vi "ArmSimulatorReal.vi"() -> ()   [LabVIEW 2020]
uses:
  <vilib>/robotics/Kinematics/Plotting/NI_Robotics_3DKinematics.lvlib
  <vilib>/picture/3D Picture Control/NI_3D Picture Control.lvlib
  <vilib>/picture/3D Picture Control/Object/Add Object (no reference).vi
  <vilib>/robotics/Kinematics/NI_Kinematics.lvlib
  <vilib>/Utility/miscctls.llb/LV3DPointTypeDef.ctl
  a5137bdd-6b26-409e-be81-2a36b3426dbb.vi
  <vilib>/robotics/Kinematics/Robot/Forward Kinematics (Point).vi
  de8be538-574b-4146-99e0-83cb54bb3f19.vi
  <vilib>/robotics/Kinematics/dyn/Gravity Loading (Point).vi
  <vilib>/picture/3D Picture Control/Object/Create Object (drawable).vi
  <vilib>/Analysis/Matrix/Datatypes/RealMatrix.ctl
  <vilib>/Analysis/Matrix/NI_Matrix.lvlib
panel:
  in  "Angle":dbl
  out "torques":dbl[](array[numeric]) format="%.2f"
  out "end effector transform":T1
  out "Steps Taken":i32
  in  "Reset 3D View":bool
  out "IK Error":errorcluster
  in  "Goal Z (in)":dbl=28.0
  in  "Goal X (in)":dbl=-33.0
  out "3D Arm Simulation":refnum<vi>(3d-picture)
  # "<-- DOWN FIELD              SCORING GRID -->"
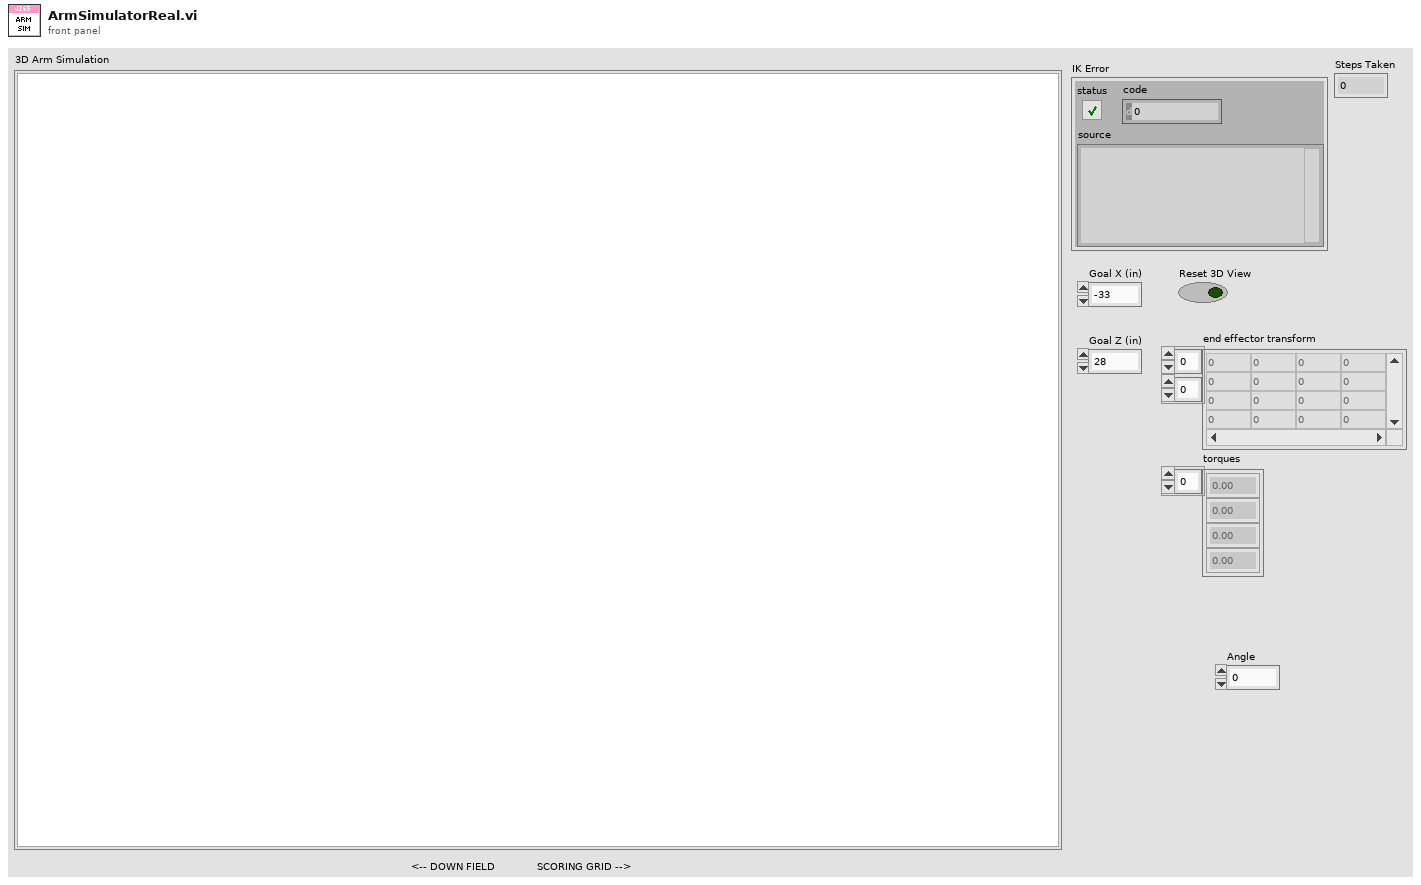
[diagram p1: front panel]
types:
  T1 = typedef "NI_Matrix.lvlib/RealMatrix.ctl" = dbl[][]
  T2 = cluster{"Red":sgl, "Green":sgl, "Blue":sgl, "Alpha":sgl}
  T3 = typedef "LV3DPointTypeDef.ctl" = cluster{"X":sgl, "Y":sgl, "Z":sgl}
  T4 = cluster{"Goal X (in)":dbl, "Goal Y (in)":dbl, "Goal Z (in)":dbl}
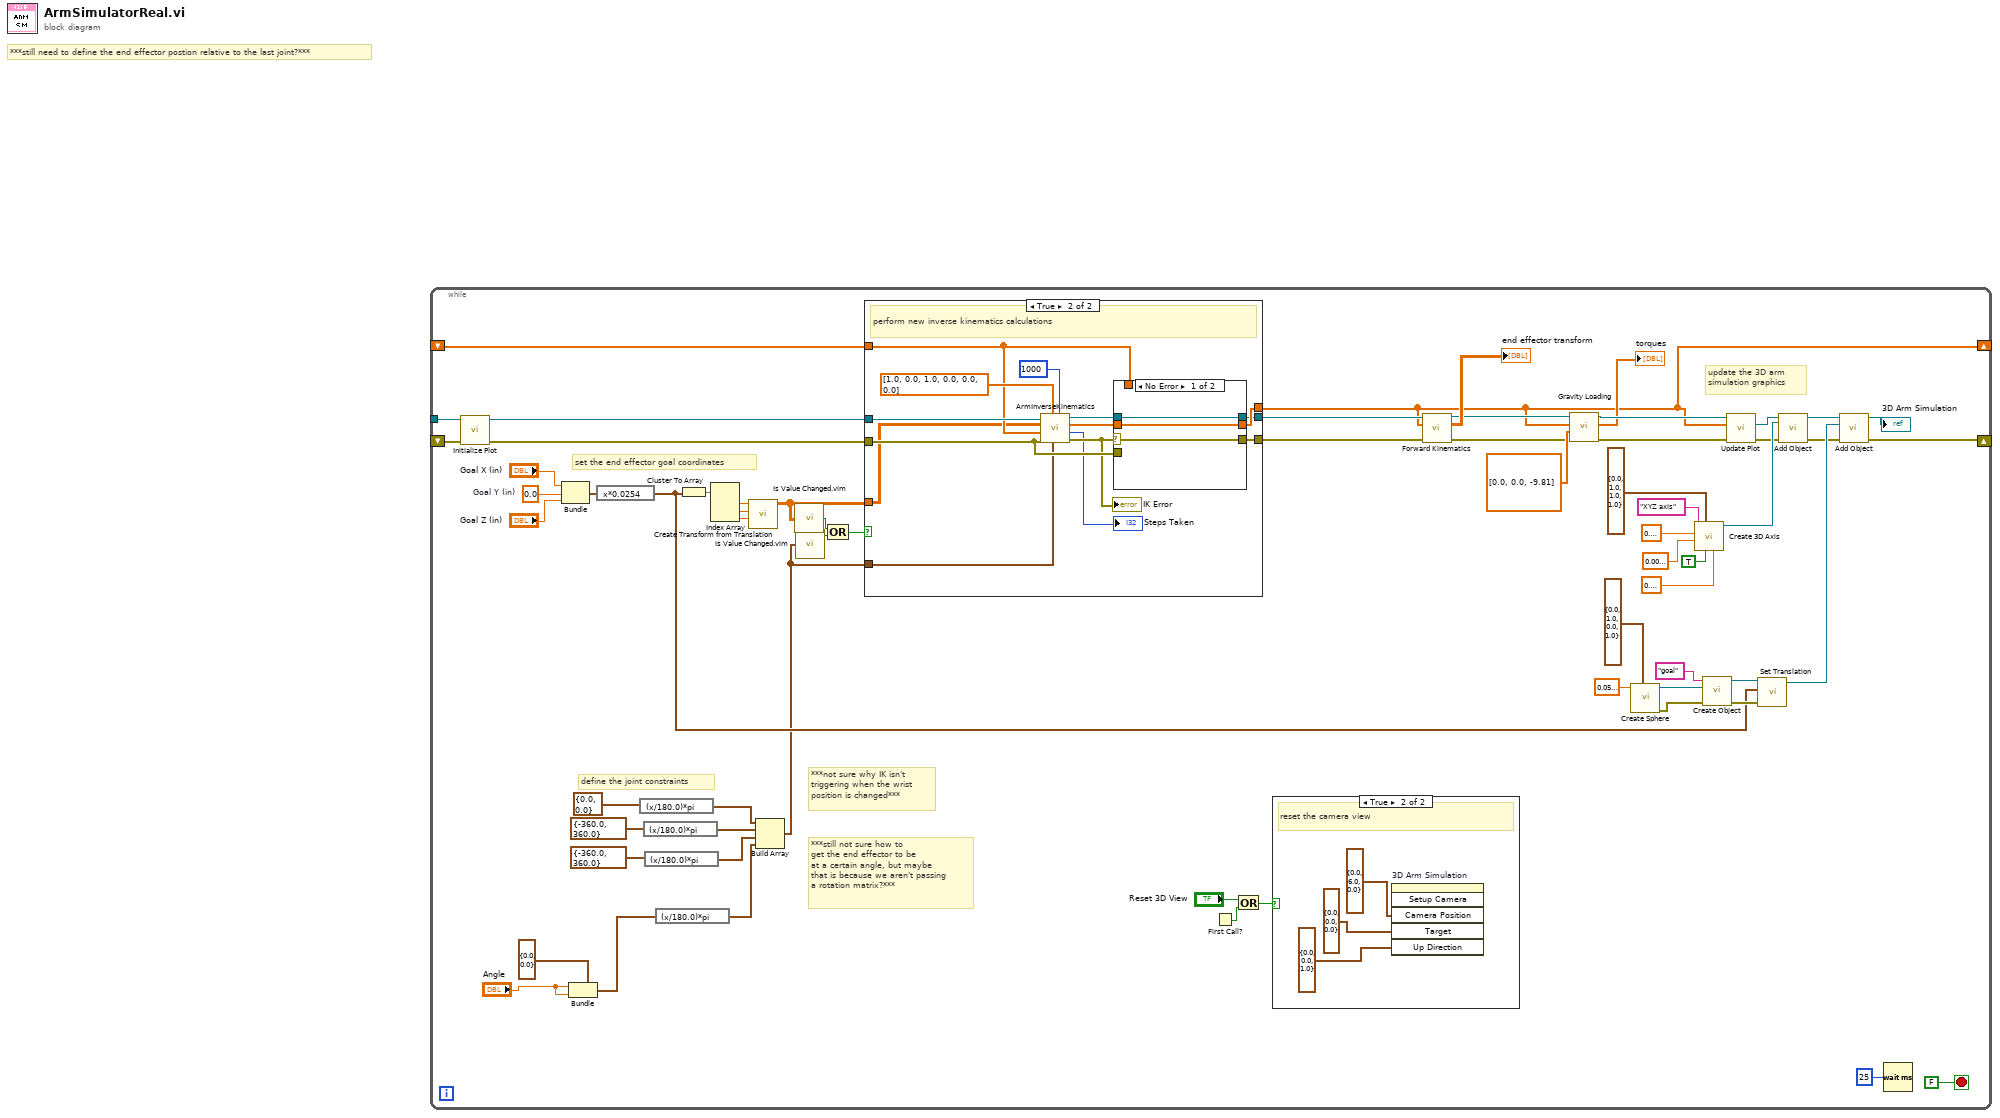
[diagram p0: block diagram]
diagram:
  # "***still need to define the end effector postion relative to the last joint?***"
  n1 = while {
    tunnel: _ -> [w50]
    shift-right: [w2] -> _
    shift-left: _ -> [w32]
    shift-right: [w17] -> _
    shift-left: [w49] -> w1
    stop <- FALSE stop-if-true
    w45 = 0.0  # Goal Y (in)
    # "***still not sure how to\nget the end effector to be\nat a certain angle, but maybe \nthat is because we aren't passing\na rotation matrix?***"
    # "***not sure why IK isn't\ntriggering when the wrist\nposition is changed***"
    # "define the joint constraints"
    # "set the end effector goal coordinates"
    # "update the 3D arm\nsimulation graphics"
    n2 = call <vilib>:"Initialize Plot.vi"("error in (no error)"=w49, "serial arm in"=w50) -> ("error out"=w43:errorcluster, "serial arm out"=w40:refnum<class "NI_Robotics_Serial Robot Arm.lvclass">)  [unwired: 8 in]
    n3 = Bundle("Goal X (in)"="Goal X (in)", "Goal Y (in)"=w45, "Goal Z (in)"="Goal Z (in)") -> (w42:T4)  [unwired: 1 in]
    n4 = Bundle(cluster=cluster{"Angle":dbl, "Angle":dbl} {"Angle"=0.0, "Angle"=0.0}, "Angle"="Angle", "Angle"="Angle") -> (w9:cluster{"Angle":dbl, "Angle":dbl})
    n5 = expression code="x*0.0254" ("degrees to radians")(w42) -> (w41:T4)
    n6 = expression code="(x/180.0)*pi" ("degrees to radians")(cluster{dbl, dbl} {0.0, 0.0}) -> (w12:cluster{dbl, dbl})
    n7 = expression code="(x/180.0)*pi" ("degrees to radians")(cluster{dbl, dbl} {-360.0, 360.0}) -> (w25:cluster{dbl, dbl})
    n8 = expression code="(x/180.0)*pi" ("degrees to radians")(cluster{dbl, dbl} {-360.0, 360.0}) -> (w23:cluster{dbl, dbl})
    n9 = expression code="(x/180.0)*pi" ("degrees to radians")(w9) -> (w22:cluster{"Angle":dbl, "Angle":dbl})
    n10 = Cluster To Array(cluster=w41) -> (array=w31:dbl[])
    n11 = Index Array(array=w31) -> (element #1=w35:dbl, element #2=w34:dbl, element #3=w33:dbl)  [unwired: 3 in]
    n12 = call <vilib>:"Create Transform from Translation.vi"("z"=w33, "y"=w34, "x"=w35) -> ("transform"=w30:T1)  [unwired: 8 in]
    n13 = Build Array(w12, w25, w23, w22) -> (w29:cluster{"Angle":dbl, "Angle":dbl}[])
    n14 = call "Is Value Changed.vim"("value"=w30) -> ("changed or first call?"=w27:bool)
    n15 = call "Is Value Changed.vim"("value"=w29) -> ("changed or first call?"=w28:bool)
    n16 = Compound Arithmetic op=OR(w27, w28) -> (w10:bool)
    n17 = case shown="True" w10 {
      tunnel: [w67 w81] -> w2
      tunnel: [w69 w79] -> w20
      tunnel: [w68 w78] -> w16
      tunnel: w43 -> [w68 w77]
      tunnel: w40 -> [w69 w75]
      tunnel: w32 -> [w67 w73]
      tunnel: w29 -> [_ w72]
      tunnel: w30 -> [_ w71]
      frame False {
        # "the end effector goal postion has not changed"
      }
      frame True {
        # "perform new inverse kinematics calculations"
        n18 = call "ArmInverseKinematics.vi"("max steps"=1000, "joint constraints"=w72, "mask"=dbl[] [1.0, 0.0, 1.0, 0.0, 0.0, 0.0], "error in (no error)"=w77, "current joint positions"=w73, "end effector transform"=w71, "serial arm in"=w75) -> ("error out"=w76:errorcluster, "steps taken"=→"Steps Taken":i32, "joint positions"=w82:dbl[], "serial arm out"=w80:refnum<class "NI_Robotics_Serial Robot Arm.lvclass">)  [unwired: 1 in]
        "IK Error" <- w76
        n19 = case shown="No Error" w76 {
          selector: w76 -> [w84 _]
          tunnel: w82 -> [w86 _]
          tunnel: [w86 w89] -> w81
          tunnel: w80 -> [w85 w88]
          tunnel: [w85 w88] -> w79
          tunnel: w73 -> [_ w89]
          tunnel: [w84 w87] -> w78
          tunnel: w77 -> [_ w87]
          frame No Error {
          }
          frame Error {
          }
        }
      }
    }
    n20 = First Call?() -> (First Call?: T/F=w39:bool)
    n21 = Or(x="Reset 3D View", y=w39) -> (x .or. y?=w38:bool)
    n22 = case shown="True" w38 {
      frame False {
      }
      frame True {
        # "reset the camera view"
        n23 = invoke on="3D Arm Simulation" class="SceneGraphDisp (strict)" method="Setup Camera"("Camera Position"=T3 {"X"=0.0, "Y"=6.0, "Z"=0.0}, "Target"=T3 {"X"=0.0, "Y"=0.0, "Z"=0.0}, "Up Direction"=T3 {"X"=0.0, "Y"=0.0, "Z"=1.0}) -> ()  [unwired: 3 in, 6 out]
      }
    }
    n24 = call-poly <vilib>:"Forward Kinematics.vi"("error in (no error)"=w16, "joint positions"=w2, "serial arm in"=w20) -> ("error out"=w6:errorcluster, "end effector transform"=→"end effector transform":T1, "serial arm out"=w7:refnum<class "NI_Robotics_Serial Robot Arm.lvclass">)  [unwired: 6 in]
    n25 = call-poly <vilib>:"Gravity Loading.vi"("error in (no error)"=w6, "gravity"=dbl[] [0.0, 0.0, -9.81], "joint positions"=w2, "serial arm in"=w7) -> ("error out"=w5:errorcluster, "torques"=→"torques":dbl[], "serial arm out"=w4:refnum<class "NI_Robotics_Serial Robot Arm.lvclass">)  [unwired: 5 in]
    n26 = call <vilib>:"Create Sphere.vi"("Color"=T2 {"Red"=0.0, "Green"=1.0, "Blue"=0.0, "Alpha"=1.0}, "Radius"=sgl 0.05) -> ("error out"=w15:errorcluster, "New Sphere Refnum"=w46:refnum<vi>)  [unwired: 8 in]
    n27 = call <vilib>:"Create 3D Axis.vi"("Character Size"=sgl 0.1, "Axis label?"=TRUE, "Color"=T2 {"Red"=0.0, "Green"=1.0, "Blue"=1.0, "Alpha"=1.0}, "Radius"=sgl 0.01, "Length"=sgl 0.2, "Name"="XYZ axis") -> ("New Object Refnum"=w57:refnum<vi>)  [unwired: 4 in, 1 out]
    n28 = call-poly <vilib>:"Create Object.vi"("error in (no error)"=w15, "Geometry"=w46, "Name"="goal") -> ("error out"=w54:errorcluster, "Scene:New Object"=w51:refnum<vi>)  [unwired: 7 in]
    n29 = call <vilib>:"Update Plot.vi"("error in (no error)"=w5, "joint positions"=w2, "serial arm in"=w4) -> ("error out"=w19:errorcluster, "serial arm scene"=w64:refnum<vi>)  [unwired: 6 in, 1 out]
    n30 = call <vilib>:"Set Translation.vi"("error in (no error)"=w54, "Translation"=w41, "Scene Object"=w51) -> ("Translated Object"=w55:refnum<vi>)  [unwired: 7 in, 1 out]
    n31 = call-poly <vilib>:"Add Object.vi"("error in (no error)"=w19, "New Object In"=w57, "Scene Object In"=w64) -> ("error out"=w18:errorcluster, "Scene Object Out"=w56:refnum<vi>)  [unwired: 7 in]
    n32 = call-poly <vilib>:"Add Object.vi"("error in (no error)"=w18, "New Object In"=w55, "Scene Object In"=w56) -> ("error out"=w17:errorcluster, "Scene Object Out"=→"3D Arm Simulation":refnum<vi>)  [unwired: 7 in]
    n33 = Wait (ms)(milliseconds to wait=u32 25) -> ()  [unwired: 1 out]
  }
